vi "CLC_Gen3_L1_GainPhase_ENA.vi"() -> ()   [LabVIEW 2023, in "Clover_Cell.lvlib"]
uses:
  lib/CTL/Keysight_VNA.ctl
  Clover_Cell.lvlib
  lib/Keysight/Keysight.lvlib
panel:
  in  "Waiting Time(ms)":u32=100
  in  "sParameter":i32=21
  in  "Step_Freq(GHz)":dbl=0.5 format="%#_13g"
  in  "Stop_Freq(GHz)":dbl=31.5
  in  "Start_Freq(GHz)":dbl=26.5
  in  "Polarity":u16(ring) items=["H", "V"]
  in  "TRXmode":u16(ring)=1 items=["Rx"=2, "Tx"=1]
  out "Step-2":bool
  out "PHASE 2":i32
  out "GAIN 2":i32
  out "Channel 2":i32
  out "Step-1":bool
  out "Channel":i32
  out "GAIN":i32
  out "PHASE":i32
  out "Marker_array":dbl[](array[numeric])
  out "Phase":dbl[][](graph)
  in  "FileName_Note":string
  in  "VISA resource name":refnum<visa-resource-name>="TCPIP0::192.168.100.12::inst0::INSTR"
  out "Return State":bool
  out "output cluster":T1={"address"="192.168.100.111", "remote port or service name"=5025, "timeout ms (60000)"=10000}
  out "Gain":dbl[][](graph)
  out "error out":errorcluster
  # "CLC-Gen3-L1-GainPhase-Sweep-ENA"
  # "Setting"
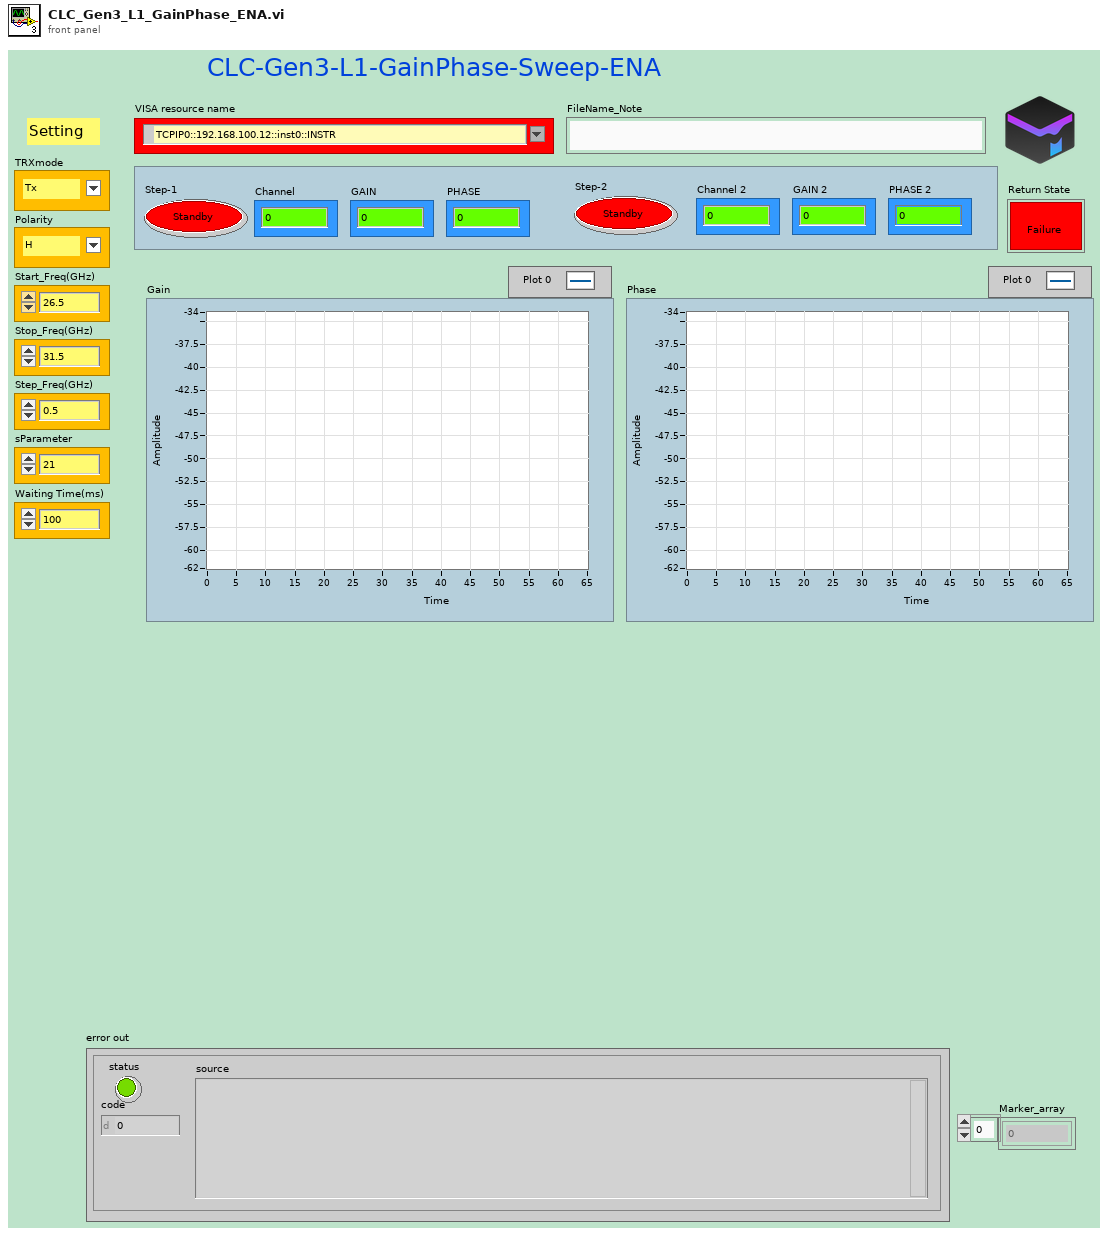
[diagram p1: front panel]
types:
  T1 = cluster{"address":string, "remote port or service name":u16, "timeout ms (60000)":i32}
  T2 = typedef "Keysight_VNA.ctl" = enum16{"Init", "queryMarker", "setSweepPoint", "setMarkerFreq", "setMeasureFormat", "setFreqStartStop", "setMarkerOnOFF", "setMarkerFormat_LOGP", "setMeasPAR_S", "setTriggerSingle", "Trigger_Save_SnP", "Trigger_Single", "Close"}
  T3 = cluster{"Mode":u16, "Polarity":u16, "CH_ON/OFF":u16, "Channel":i32, "Gain":i32, "Phase":i32}
  T4 = cluster{"setSweepPoint":i32, "Meas":i32, "Mark":i32, "Freq_GHz":dbl, "Start_Freq(GHz)":dbl, "Stop_Freq(GHz)":dbl, "sParameter":i32}
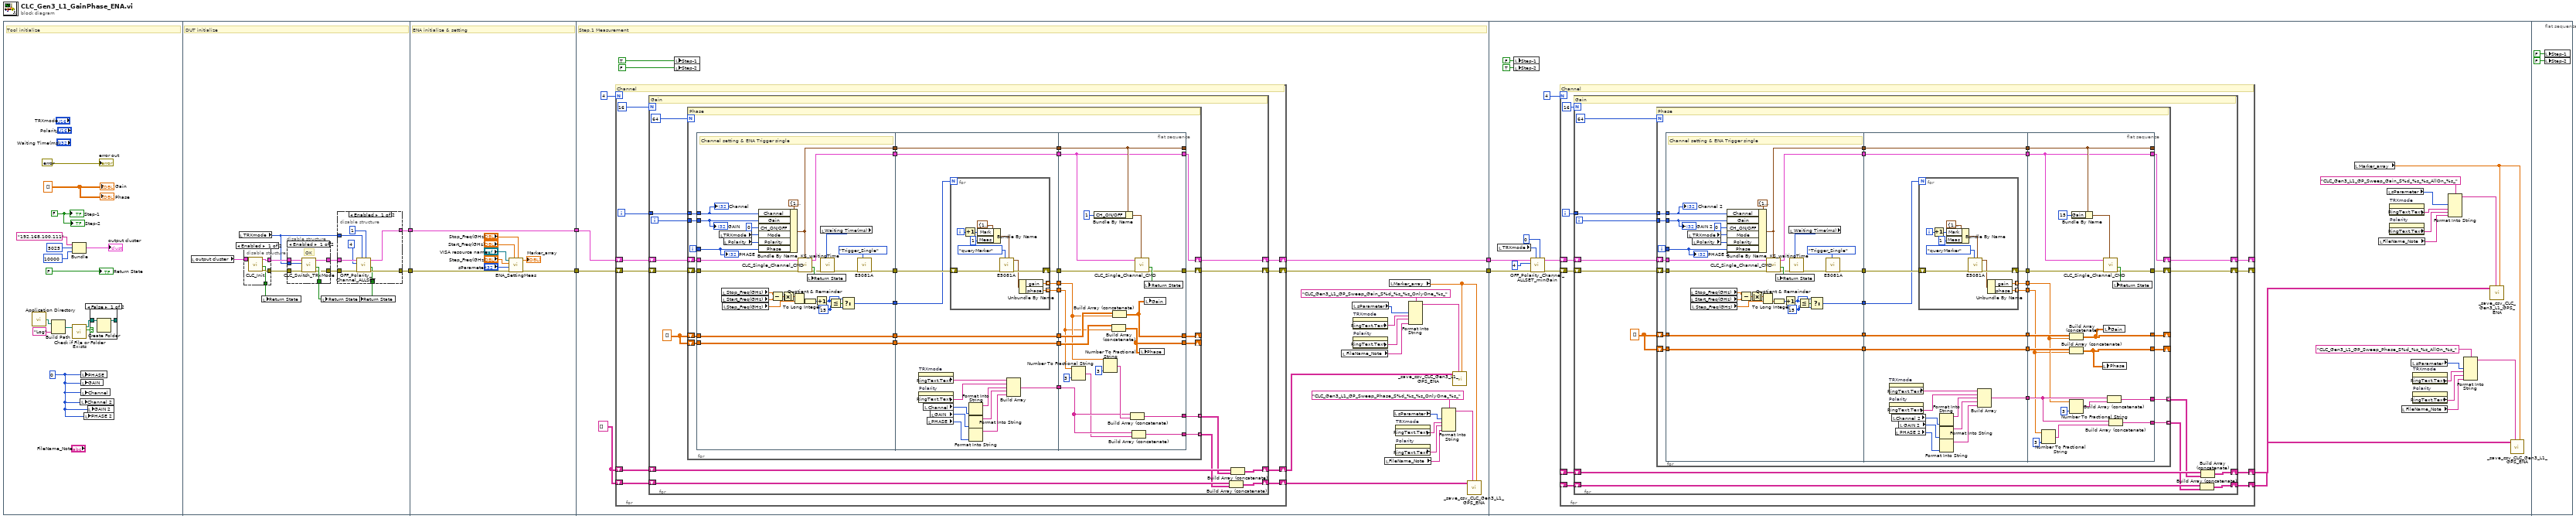
[diagram p0: block diagram]
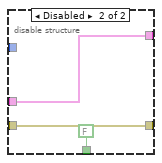
[diagram p3: hidden frame]
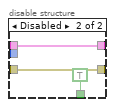
[diagram p4: hidden frame]
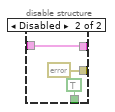
[diagram p5: hidden frame]
diagram:
  n1 = flat-sequence {
    tunnel: [w25] -> w6
    tunnel: [w29] -> w5
    tunnel: w6 -> [w70]
    tunnel: w5 -> [w63]
    tunnel: [w70] -> w4
    tunnel: [w64] -> w3
    tunnel: w4 -> [w93]
    tunnel: w3 -> [w90]
    tunnel: [w92] -> w2
    tunnel: [w91] -> w1
    tunnel: w2 -> [w244]
    tunnel: w1 -> [w245]
    frame #0 {
      w8 = FALSE ("Step-1")
      w7 = 0 ("PHASE")
      w9 = dbl[][] []
      # "Tool initialize"
      n2 = call <vilib>:"Application Directory.vi"() -> ("Application Directory"=w13:path)
      n3 = Build Path(base path=w13, name or relative path="Log") -> (appended path=w10:path)
      n4 = Bundle("address"="192.168.100.111", "remote port or service name"=u16 5025, "timeout ms (60000)"=10000) -> (→"output cluster":T1)  [unwired: 1 in]
      n5 = call <vilib>:"Check if File or Folder Exists.vi"("path"=w10) -> ("file or folder exists?"=w12:bool, "dup path"=w11:path)  [unwired: 8 in, 1 out]
      n6 = local write "Channel 2"(w7) -> ()
      n7 = local write "PHASE"(w7) -> ()
      n8 = local write "GAIN"(w7) -> ()
      n9 = local write "Channel"(w7) -> ()
      n10 = local write "PHASE 2"(w7) -> ()
      n11 = local write "GAIN 2"(w7) -> ()
      n12 = case shown="False" w12 {
        tunnel: w11 -> [w22 w23]
        tunnel: [w21 w23] -> _
        frame False {
          n13 = Create Folder(path (use dialog)=w22) -> (created path=w21:path)  [unwired: 2 in, 2 out]
        }
        frame True {
        }
      }
      "error out" <- errorcluster {"status"=FALSE, "code"=0, "source"=""} ("error out")
      "Return State" <- FALSE ("OK?")
      "Gain" <- w9
      "Phase" <- w9
      "Step-1" <- w8
      "Step-2" <- w8
    }
    frame #1 {
      # "DUT initialize"
      n14 = local read "output cluster"() -> (w34:T1)
      n15 = local read "TRXmode"() -> (w24:u16)
      n16 = disable-structure shown="Enabled" {
        disable-tunnel: w34 -> [w58 w61]
        disable-tunnel: [w57 w61] -> w33
        disable-tunnel: [w56 errorcluster {"status"=FALSE, "code"=0, "source"=""} ("error in (no error)")] -> w31
        disable-tunnel: [w55 TRUE ("OK?")] -> w26
        frame Enabled {
          n17 = call "CLC_Init.vi"("TCPIPin"=w58) -> ("error out"=w56:errorcluster, "Status"=w55:bool, "TCPIPin 2"=w57:T1)  [unwired: 8 in]
        }
        frame Disabled {
        }
      }
      n18 = local write "Return State"(w26) -> ()
      n19 = disable-structure shown="Enabled" {
        disable-tunnel: w33 -> [w51 w53]
        disable-tunnel: [w50 TRUE ("OK?")] -> w32
        disable-tunnel: w31 -> [w49 w52]
        disable-tunnel: [w48 w52] -> w30
        disable-tunnel: [w47 w53] -> w28
        disable-tunnel: w24 -> [w46 _]
        frame Enabled {
          # "OK"
          n20 = call "CLC_Switch_TRxMode.vi"("error in (no error)"=w49, "Text Ring"=w46, "TCPIPin"=w51) -> ("error out"=w48:errorcluster, "OK?"=w50:bool, "TCPIPin 2"=w47:T1)  [unwired: 6 in]
        }
        frame Disabled {
        }
      }
      n21 = local write "Return State"(w32) -> ()
      n22 = disable-structure shown="Enabled" {
        disable-tunnel: w30 -> [w42 w44]
        disable-tunnel: [w41 w44] -> w29
        disable-tunnel: w28 -> [w40 w43]
        disable-tunnel: [w39 FALSE ("OK?")] -> w27
        disable-tunnel: w24 -> [w37 _]
        disable-tunnel: [w35 w43] -> w25
        frame Enabled {
          n23 = call "OFF_Polarity_Channel_ALLSET.vi"("CH_ON:0/OFF:1"=u16 1, "Mode"=w37, "error in"=w42, "Channel"=4, "TCPIPin"=w40) -> ("error out"=w41:errorcluster, "OK?"=w39:bool, "TCPIPout"=w35:T1)  [unwired: 4 in]
        }
        frame Disabled {
        }
      }
      n24 = local write "Return State"(w27) -> ()
    }
    frame #2 {
      # "ENA initialize & setting"
      n25 = call "ENA_SettingMeas.vi"("Stop_Freq(GHz)"="Stop_Freq(GHz)", "Start_Freq(GHz)"="Start_Freq(GHz)", "error in"=w63, "sParameter"="sParameter", "Step_Freq(GHz)"="Step_Freq(GHz)", "VISA IN"="VISA resource name") -> ("error out"=w64:errorcluster, "Marker_array"=→"Marker_array":dbl[])  [unwired: 4 in]
    }
    frame #3 {
      w88 = string[][] []
      # "Step.1 Measurement"
      n26 = for {
        N: 4 -> [_]
        shift-right: [w102] -> w92
        shift-left: w93 -> [w103]
        shift-right: [w101] -> w91
        shift-left: w90 -> [w100]
        shift-right: [w95] -> w87
        shift-left: w88 -> [w97]
        shift-right: [w94] -> w86
        shift-left: w88 -> [w96]
        i -> [w98]
        # "Channel"
        n27 = for {
          N: 16 -> [_]
          shift-right: [w116] -> w102
          shift-left: w103 -> [w117]
          shift-right: [w115] -> w101
          shift-left: w100 -> [w114]
          tunnel: w98 -> [w112]
          shift-right: [w106] -> w95
          shift-left: w97 -> [w110]
          shift-right: [w105] -> w94
          shift-left: w96 -> [w109]
          i -> [w111]
          w104 = dbl[][] []
          # "Gain"
          n28 = for {
            N: 64 -> [_]
            shift-right: [w132] -> w116
            shift-left: w117 -> [w144]
            shift-right: [w131] -> w115
            shift-left: w114 -> [w143]
            tunnel: w112 -> [w142]
            tunnel: w111 -> [w141]
            tunnel: [w127] -> w108 mode=indexing
            tunnel: [w126] -> w107 mode=indexing
            shift-right: [w119] -> _
            shift-left: w104 -> [w123]
            shift-right: [w118] -> _
            shift-left: w104 -> [w120]
            i -> [w140]
            # "Phase"
            n29 = flat-sequence {
              tunnel: w144 -> [w172]
              tunnel: w143 -> [w171]
              tunnel: w142 -> [w170]
              tunnel: w141 -> [w167]
              tunnel: w140 -> [w161]
              tunnel: [w163] -> w139
              tunnel: [w150] -> w138
              tunnel: [w149] -> w137
              tunnel: [w148] -> w136
              tunnel: [w146] -> w124
              tunnel: w123 -> [w146]
              tunnel: [w145] -> w121
              tunnel: w120 -> [w145]
              tunnel: w139 -> [w191]
              tunnel: w138 -> [w190]
              tunnel: w137 -> [w189]
              tunnel: w136 -> [w188]
              tunnel: [w192] -> w135
              tunnel: [w190] -> w134
              tunnel: [w189] -> w133
              tunnel: [w187] -> w130
              tunnel: [w186] -> w129
              tunnel: [w177] -> w128
              tunnel: [w176] -> w125
              tunnel: w124 -> [w176]
              tunnel: [w175] -> w122
              tunnel: w121 -> [w175]
              tunnel: [w220] -> _
              tunnel: [w217] -> w132
              tunnel: [w222] -> w131
              tunnel: w135 -> [w221]
              tunnel: w134 -> [w217]
              tunnel: w133 -> [w220]
              tunnel: w130 -> [w207]
              tunnel: w129 -> [w206]
              tunnel: w128 -> [w213]
              tunnel: [w211] -> w127
              tunnel: [w210] -> w126
              tunnel: w125 -> [w209]
              tunnel: w122 -> [w208]
              tunnel: [w205] -> w119
              tunnel: [w204] -> w118
              frame #0 {
                w160 = 15 ("y")
                # "Channel setting & ENA Trigger single"
                n30 = local read "TRXmode"() -> (w168:u16)
                n31 = local read "Stop_Freq(GHz)"() -> (w153:dbl)
                n32 = local read "Start_Freq(GHz)"() -> (w152:dbl)
                n33 = local read "Step_Freq(GHz)"() -> (w151:dbl)
                n34 = local read "Polarity"() -> (w169:u16)
                n35 = Bundle By Name(cluster=T3 {"Mode"=1, "Polarity"=1, "CH_ON/OFF"=1, "Channel"=0, "Gain"=0, "Phase"=0} ("Channel params"), "Channel"=w170, "Gain"=w167, "CH_ON/OFF"=u16 0, "Mode"=w168, "Polarity"=w169, "Phase"=w161) -> (w149:T3)
                n36 = Subtract(x=w153, y=w152) -> (x-y=w159:dbl)
                n37 = Absolute Value(x=w159) -> (abs(x)=w158:dbl)
                n38 = Quotient & Remainder(x=w158, y=w151) -> (floor(x/y)=w157:dbl)  [unwired: 1 out]
                n39 = call "CLC_Single_Channel_CMD.vi"("Channel params"=w149, "error in"=w171, "TCPIPin"=w172) -> ("error out"=w166:errorcluster, "OK?"=w173:bool, "TCPIPout"=w150:T1)  [unwired: 6 in]
                n40 = To Long Integer(number=w157) -> (32bit integer=w156:i32)
                n41 = local write "Return State"(w173) -> ()
                n42 = Increment(x=w156) -> (x+1=w154:i32)
                n43 = local read "Waiting Time(ms)"() -> (w147:u32)
                n44 = call "KS_waitingTime.vi"("Waiting Time(ms)"=w147, "error in"=w166) -> ("error out"=w164:errorcluster)  [unwired: 9 in]
                n45 = Less Or Equal?(x=w154, y=w160) -> (x <= y?=w155:bool)
                n46 = Select(t=w154, s=w155, f=w160) -> (s? t:f=w148:i32)
                n47 = call "E5081A.vi"("Function_VNA"=Keysight_VNA."Trigger_Single", "error in"=w164) -> ("error out"=w163:errorcluster)  [unwired: 8 in, 1 out]
                "PHASE" <- w161
                "GAIN" <- w167
                "Channel" <- w170
              }
              frame #1 {
                n48 = property on="TRXmode" class="Ring (strict)"() -> ("RingText.Text"=w182:string)  [unwired: 2 in, 2 out]
                n49 = property on="Polarity" class="Ring (strict)"() -> ("RingText.Text"=w181:string)  [unwired: 2 in, 2 out]
                n50 = local read "Channel"() -> (w185:i32)
                n51 = local read "PHASE"() -> (w183:i32)
                n52 = local read "GAIN"() -> (w184:i32)
                n53 = for {
                  N: w188 -> [_]
                  shift-right: [w202] -> w192
                  shift-left: w191 -> [w203]
                  tunnel: [w194] -> w187 mode=indexing
                  tunnel: [w193] -> w186 mode=indexing
                  i -> [w199]
                  n54 = Increment(x=w199) -> (x+1=w197:i32)
                  n55 = Bundle By Name(cluster=T4 {"setSweepPoint"=11, "Meas"=1, "Mark"=0, "Freq_GHz"=0.0, "Start_Freq(GHz)"=0.0, "Stop_Freq(GHz)"=0.0, "sParameter"=1} ("Input"), "Mark"=w197, "Meas"=1) -> (w196:T4)
                  n56 = call "E5081A.vi"("Input"=w196, "Function_VNA"=Keysight_VNA."queryMarker", "error in"=w203) -> ("error out"=w202:errorcluster, "queryMarker"=w195:cluster{"gain":dbl, "phase":dbl})  [unwired: 7 in]
                  n57 = Unbundle By Name(w195) -> ("gain"=w194:dbl, "phase"=w193:dbl)
                }
                n58 = Format Into String(w185) -> (resulting string=w180:string)  [unwired: 3 in, 1 out]
                n59 = Format Into String(w184) -> (resulting string=w179:string)  [unwired: 3 in, 1 out]
                n60 = Format Into String(w183) -> (resulting string=w178:string)  [unwired: 3 in, 1 out]
                n61 = Build Array(w182, w181, w180, w179, w178) -> (w177:string[])
              }
              frame #2 {
                n62 = Number To Fractional String(number=w206, precision (6)=i16 3) -> (F-format string=w212:string[])  [unwired: 2 in]
                n63 = Bundle By Name(cluster=w220, "CH_ON/OFF"=u16 1) -> (w218:T3)
                n64 = Number To Fractional String(number=w207, precision (6)=i16 3) -> (F-format string=w214:string[])  [unwired: 2 in]
                n65 = Build Array (concatenate)(w208, w206) -> (w204:dbl[][])
                n66 = Build Array (concatenate)(w209, w207) -> (w205:dbl[][])
                n67 = Build Array (concatenate)(w213, w214) -> (w211:string[])
                n68 = Build Array (concatenate)(w213, w212) -> (w210:string[])
                n69 = call "CLC_Single_Channel_CMD.vi"("Channel params"=w218, "error in"=w221, "TCPIPin"=w217) -> ("error out"=w222:errorcluster, "OK?"=w223:bool)  [unwired: 6 in, 1 out]
                n70 = local write "Phase"(w204) -> ()
                n71 = local write "Return State"(w223) -> ()
                n72 = local write "Gain"(w205) -> ()
              }
            }
          }
          n73 = Build Array (concatenate)(w109, w107) -> (w105:string[][])
          n74 = Build Array (concatenate)(w110, w108) -> (w106:string[][])
        }
      }
      n75 = local write "Step-1"(TRUE ("Step-1")) -> ()
      n76 = local write "Step-2"(FALSE ("Step-2")) -> ()
      n77 = local read "FileName_Note"() -> (w74:string)
      n78 = local read "sParameter"() -> (w77:i32)
      n79 = property on="TRXmode" class="Ring (strict)"() -> ("RingText.Text"=w76:string)  [unwired: 2 in, 2 out]
      n80 = property on="Polarity" class="Ring (strict)"() -> ("RingText.Text"=w75:string)  [unwired: 2 in, 2 out]
      n81 = local read "FileName_Note"() -> (w71:string)
      n82 = local read "Marker_array"() -> (w85:dbl[])
      n83 = local read "sParameter"() -> (w82:i32)
      n84 = property on="TRXmode" class="Ring (strict)"() -> ("RingText.Text"=w73:string)  [unwired: 2 in, 2 out]
      n85 = property on="Polarity" class="Ring (strict)"() -> ("RingText.Text"=w72:string)  [unwired: 2 in, 2 out]
      n86 = Format Into String(format string="CLC_Gen3_L1_GP_Sweep_Gain_S%d_%s_%s_OnlyOne_%s_" ("NoteName"), w77, w76, w75, w74) -> (resulting string=w83:string)  [unwired: 2 in, 1 out]
      n87 = Format Into String(format string="CLC_Gen3_L1_GP_Sweep_Phase_S%d_%s_%s_OnlyOne_%s_" ("NoteName"), w82, w73, w72, w71) -> (resulting string=w80:string)  [unwired: 2 in, 1 out]
      n88 = call "_save_csv_CLC_Gen3_L1_GPS_ENA.vi"("Marker_array"=w85, "NoteName"=w83, "array in"=w87) -> ()  [unwired: 8 in, 1 out]
      n89 = call "_save_csv_CLC_Gen3_L1_GPS_ENA.vi"("Marker_array"=w85, "NoteName"=w80, "array in"=w86) -> ()  [unwired: 8 in, 1 out]
    }
    frame #4 {
      n90 = local read "TRXmode"() -> (w242:u16)
      n91 = local write "Step-1"(FALSE ("Step-1")) -> ()
      n92 = local write "Step-2"(TRUE ("Step-2")) -> ()
      n93 = call "OFF_Polarity_Channel_ALLSET_minGain.vi"("CH_ON:0/OFF:1"=u16 0, "Mode"=w242, "error in"=w245, "Channel"=4, "TCPIPin"=w244) -> ("error out"=w246:errorcluster, "TCPIPout"=w247:T1)  [unwired: 4 in, 1 out]
      n94 = for {
        N: 4 -> [_]
        shift-right: [w257] -> _
        shift-left: w247 -> [w258]
        shift-right: [w256] -> _
        shift-left: w246 -> [w255]
        shift-right: [w250] -> w234
        shift-left: _ -> [w252]
        shift-right: [w249] -> w233
        shift-left: _ -> [w251]
        i -> [w253]
        # "Channel"
        n95 = for {
          N: 16 -> [_]
          shift-right: [w271] -> w257
          shift-left: w258 -> [w272]
          shift-right: [w270] -> w256
          shift-left: w255 -> [w269]
          tunnel: w253 -> [w267]
          shift-right: [w261] -> w250
          shift-left: w252 -> [w265]
          shift-right: [w260] -> w249
          shift-left: w251 -> [w264]
          i -> [w266]
          w259 = dbl[][] []
          # "Gain"
          n96 = for {
            N: 64 -> [_]
            shift-right: [w287] -> w271
            shift-left: w272 -> [w299]
            shift-right: [w286] -> w270
            shift-left: w269 -> [w298]
            tunnel: w267 -> [w297]
            tunnel: w266 -> [w296]
            tunnel: [w282] -> w263 mode=indexing
            tunnel: [w281] -> w262 mode=indexing
            shift-right: [w274] -> _
            shift-left: w259 -> [w278]
            shift-right: [w273] -> _
            shift-left: w259 -> [w275]
            i -> [w295]
            # "Phase"
            n97 = flat-sequence {
              tunnel: w299 -> [w327]
              tunnel: w298 -> [w326]
              tunnel: w297 -> [w325]
              tunnel: w296 -> [w322]
              tunnel: w295 -> [w316]
              tunnel: [w318] -> w294
              tunnel: [w305] -> w293
              tunnel: [w304] -> w292
              tunnel: [w303] -> w291
              tunnel: [w301] -> w279
              tunnel: w278 -> [w301]
              tunnel: [w300] -> w276
              tunnel: w275 -> [w300]
              tunnel: w294 -> [w346]
              tunnel: w293 -> [w345]
              tunnel: w292 -> [w344]
              tunnel: w291 -> [w343]
              tunnel: [w347] -> w290
              tunnel: [w345] -> w289
              tunnel: [w344] -> w288
              tunnel: [w342] -> w285
              tunnel: [w341] -> w284
              tunnel: [w332] -> w283
              tunnel: [w331] -> w280
              tunnel: w279 -> [w331]
              tunnel: [w330] -> w277
              tunnel: w276 -> [w330]
              tunnel: [w375] -> _
              tunnel: [w373] -> w287
              tunnel: [w377] -> w286
              tunnel: w290 -> [w376]
              tunnel: w289 -> [w373]
              tunnel: w288 -> [w375]
              tunnel: w285 -> [w362]
              tunnel: w284 -> [w359]
              tunnel: w283 -> [w369]
              tunnel: [w367] -> w282
              tunnel: [w366] -> w281
              tunnel: w280 -> [w364]
              tunnel: w277 -> [w363]
              tunnel: [w361] -> w274
              tunnel: [w360] -> w273
              frame #0 {
                w315 = 15 ("y")
                # "Channel setting & ENA Trigger single"
                n98 = local read "TRXmode"() -> (w323:u16)
                n99 = local read "Stop_Freq(GHz)"() -> (w308:dbl)
                n100 = local read "Start_Freq(GHz)"() -> (w307:dbl)
                n101 = local read "Step_Freq(GHz)"() -> (w306:dbl)
                n102 = local read "Polarity"() -> (w324:u16)
                n103 = Bundle By Name(cluster=T3 {"Mode"=1, "Polarity"=1, "CH_ON/OFF"=1, "Channel"=0, "Gain"=0, "Phase"=0} ("Channel params"), "Channel"=w325, "Gain"=w322, "CH_ON/OFF"=u16 0, "Mode"=w323, "Polarity"=w324, "Phase"=w316) -> (w304:T3)
                n104 = Subtract(x=w308, y=w307) -> (x-y=w314:dbl)
                n105 = Absolute Value(x=w314) -> (abs(x)=w313:dbl)
                n106 = Quotient & Remainder(x=w313, y=w306) -> (floor(x/y)=w312:dbl)  [unwired: 1 out]
                n107 = call "CLC_Single_Channel_CMD.vi"("Channel params"=w304, "error in"=w326, "TCPIPin"=w327) -> ("error out"=w321:errorcluster, "OK?"=w328:bool, "TCPIPout"=w305:T1)  [unwired: 6 in]
                n108 = To Long Integer(number=w312) -> (32bit integer=w311:i32)
                n109 = local write "Return State"(w328) -> ()
                n110 = Increment(x=w311) -> (x+1=w309:i32)
                n111 = local read "Waiting Time(ms)"() -> (w302:u32)
                n112 = call "KS_waitingTime.vi"("Waiting Time(ms)"=w302, "error in"=w321) -> ("error out"=w319:errorcluster)  [unwired: 9 in]
                n113 = Less Or Equal?(x=w309, y=w315) -> (x <= y?=w310:bool)
                n114 = Select(t=w309, s=w310, f=w315) -> (s? t:f=w303:i32)
                n115 = call "E5081A.vi"("Function_VNA"=Keysight_VNA."Trigger_Single", "error in"=w319) -> ("error out"=w318:errorcluster)  [unwired: 8 in, 1 out]
                "PHASE 2" <- w316
                "GAIN 2" <- w322
                "Channel 2" <- w325
              }
              frame #1 {
                n116 = property on="TRXmode" class="Ring (strict)"() -> ("RingText.Text"=w337:string)  [unwired: 2 in, 2 out]
                n117 = property on="Polarity" class="Ring (strict)"() -> ("RingText.Text"=w336:string)  [unwired: 2 in, 2 out]
                n118 = local read "Channel 2"() -> (w340:i32)
                n119 = local read "PHASE 2"() -> (w338:i32)
                n120 = local read "GAIN 2"() -> (w339:i32)
                n121 = for {
                  N: w343 -> [_]
                  shift-right: [w357] -> w347
                  shift-left: w346 -> [w358]
                  tunnel: [w349] -> w342 mode=indexing
                  tunnel: [w348] -> w341 mode=indexing
                  i -> [w354]
                  n122 = Increment(x=w354) -> (x+1=w352:i32)
                  n123 = Bundle By Name(cluster=T4 {"setSweepPoint"=11, "Meas"=1, "Mark"=0, "Freq_GHz"=0.0, "Start_Freq(GHz)"=0.0, "Stop_Freq(GHz)"=0.0, "sParameter"=1} ("Input"), "Mark"=w352, "Meas"=1) -> (w351:T4)
                  n124 = call "E5081A.vi"("Input"=w351, "Function_VNA"=Keysight_VNA."queryMarker", "error in"=w358) -> ("error out"=w357:errorcluster, "queryMarker"=w350:cluster{"gain":dbl, "phase":dbl})  [unwired: 7 in]
                  n125 = Unbundle By Name(w350) -> ("gain"=w349:dbl, "phase"=w348:dbl)
                }
                n126 = Format Into String(w340) -> (resulting string=w335:string)  [unwired: 3 in, 1 out]
                n127 = Format Into String(w339) -> (resulting string=w334:string)  [unwired: 3 in, 1 out]
                n128 = Format Into String(w338) -> (resulting string=w333:string)  [unwired: 3 in, 1 out]
                n129 = Build Array(w337, w336, w335, w334, w333) -> (w332:string[])
              }
              frame #2 {
                n130 = Number To Fractional String(number=w359, precision (6)=i16 3) -> (F-format string=w368:string[])  [unwired: 2 in]
                n131 = Build Array (concatenate)(w363, w359) -> (w360:dbl[][])
                n132 = Number To Fractional String(number=w362, precision (6)=i16 3) -> (F-format string=w370:string[])  [unwired: 2 in]
                n133 = Build Array (concatenate)(w364, w362) -> (w361:dbl[][])
                n134 = Bundle By Name(cluster=w375, "Gain"=15) -> (w374:T3)
                n135 = local write "Phase"(w360) -> ()
                n136 = call "CLC_Single_Channel_CMD.vi"("Channel params"=w374, "error in"=w376, "TCPIPin"=w373) -> ("error out"=w377:errorcluster, "OK?"=w378:bool)  [unwired: 6 in, 1 out]
                n137 = local write "Gain"(w361) -> ()
                n138 = Build Array (concatenate)(w369, w370) -> (w367:string[])
                n139 = Build Array (concatenate)(w369, w368) -> (w366:string[])
                n140 = local write "Return State"(w378) -> ()
              }
            }
          }
          n141 = Build Array (concatenate)(w264, w262) -> (w260:string[][])
          n142 = Build Array (concatenate)(w265, w263) -> (w261:string[][])
        }
      }
      n143 = local read "Marker_array"() -> (w240:dbl[])
      n144 = local read "FileName_Note"() -> (w227:string)
      n145 = local read "sParameter"() -> (w230:i32)
      n146 = property on="TRXmode" class="Ring (strict)"() -> ("RingText.Text"=w229:string)  [unwired: 2 in, 2 out]
      n147 = property on="Polarity" class="Ring (strict)"() -> ("RingText.Text"=w228:string)  [unwired: 2 in, 2 out]
      n148 = local read "FileName_Note"() -> (w224:string)
      n149 = local read "sParameter"() -> (w238:i32)
      n150 = property on="TRXmode" class="Ring (strict)"() -> ("RingText.Text"=w226:string)  [unwired: 2 in, 2 out]
      n151 = property on="Polarity" class="Ring (strict)"() -> ("RingText.Text"=w225:string)  [unwired: 2 in, 2 out]
      n152 = Format Into String(format string="CLC_Gen3_L1_GP_Sweep_Gain_S%d_%s_%s_AllOn_%s_" ("NoteName"), w230, w229, w228, w227) -> (resulting string=w239:string)  [unwired: 2 in, 1 out]
      n153 = Format Into String(format string="CLC_Gen3_L1_GP_Sweep_Phase_S%d_%s_%s_AllOn_%s_" ("NoteName"), w238, w226, w225, w224) -> (resulting string=w237:string)  [unwired: 2 in, 1 out]
      n154 = call "_save_csv_CLC_Gen3_L1_GPS_ENA.vi"("Marker_array"=w240, "NoteName"=w239, "array in"=w234) -> ()  [unwired: 8 in, 1 out]
      n155 = call "_save_csv_CLC_Gen3_L1_GPS_ENA.vi"("Marker_array"=w240, "NoteName"=w237, "array in"=w233) -> ()  [unwired: 8 in, 1 out]
    }
    frame #5 {
      n156 = local write "Step-1"(FALSE ("Step-1")) -> ()
      n157 = local write "Step-2"(FALSE ("Step-2")) -> ()
    }
  }
